vi "initialize.vi"(0 "HGF_DSCMonitor":refnum<class "HGF_DSCMonitor.lvclass">, 3 "initializationData":variant, 5 "error in (no error)":errorcluster, 7 "binaryString":string, 8 "I8 Array":i8[](array[numeric]), 9 "prependSize? (T)":bool, 11 "byteOrder (0:big-endian, network order)":T1(ring)) -> (14 "dup HGF_DSCMonitor":refnum<class "HGF_DSCMonitor.lvclass">, 17 "found?":bool, 19 "error out":errorcluster)   [LabVIEW 2012, in "HGF_DSC.lvlib" / "HGF_DSCMonitor.lvclass"]
doc: "This is a dynamic dispatch VI to be implemented by child classes to initialize their attributes.\n\n<B>Recommendation:</B> Use Variant for initialization data."
uses:
  HGF_DSCMonitor.lvclass
  HGF_SV/HGF_Monitor/HGF_Monitor.lvclass
  HGF_DSCMonitor.lvclass/HGF_DSCMonitor.ctl
  <vilib>/lvdsc/NI_DSC.lvlib
  HGF_BaseClasses/HGF_Factory/HGF_Factory.lvclass
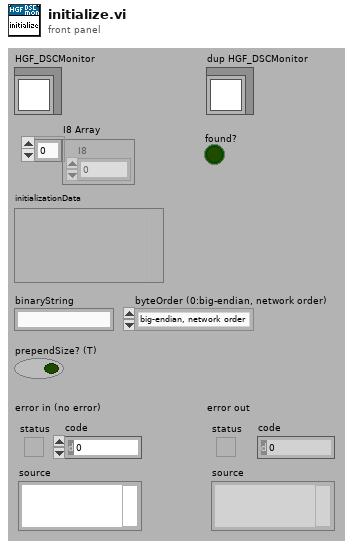
[diagram p1: front panel]
types:
  T1 = enum16{"big-endian, network order", "native, host order", "little-endian"}
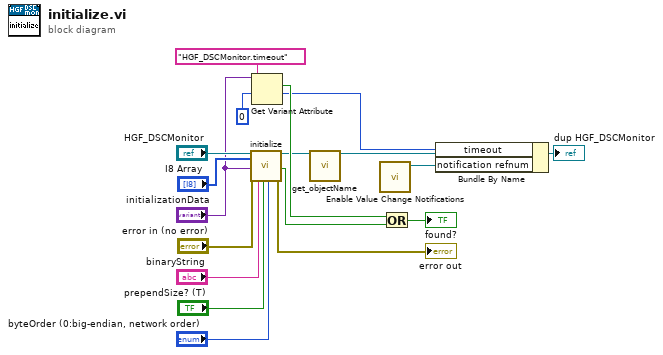
[diagram p0: block diagram]
diagram:
  n1 = call-parent "initialize.vi"("HGF_Base"="HGF_DSCMonitor", "initializationData"="initializationData", "error in (no error)"="error in (no error)", "binaryString"="binaryString", "I8 Array"="I8 Array", "prependSize? (T)"="prependSize? (T)", "byteOrder (0:big-endian, network order)"="byteOrder (0:big-endian, network order)") -> ("dup HGF_Base"=w2:refnum<class "HGF_DSCMonitor.lvclass">, "found?"=w12:bool, "error out"=→"error out":errorcluster)  [unwired: 10 out]
  n2 = Get Variant Attribute(Variant="initializationData", name="HGF_DSCMonitor.timeout", default value (empty Variant)=0) -> (found=w6:bool, value=w5:i32)  [unwired: 1 in, 2 out]
  n3 = call "get_objectName.vi"("HGF_Factory"=w2) -> ("dup HGF_Factory"=w1:refnum<class "HGF_DSCMonitor.lvclass">)  [unwired: 1 in, 17 out]
  n4 = call <vilib>:"Enable Value Change Notifications.vi"() -> ("shared variable value change notification"=w3:refnum<user-event>)  [unwired: 1 in, 10 out]
  n5 = Or(x=w6, y=w12) -> (x .or. y?=→"found?":bool)
  n6 = Bundle By Name(cluster=w1, "timeout"=w5, "notification refnum"=w3) -> (→"dup HGF_DSCMonitor":refnum<class "HGF_DSCMonitor.lvclass">)
